vi "LVClass_CorrectionDataManager ComputeDeltaCmdFromDeltaSWithCLSmooth.vi"(0 "CorrectionDataManager in":refnum<class "CorrectionDataManager.lvclass">, 5 "Delta Slopes IN":refnum<class "HasoSlopes.lvclass">, 7 "Gain in":dbl min=0.0 max=1.0, 9 "ClosedLoopSmoothing in":refnum<class "ClosedLoopSmoothing.lvclass">, 11 "error in (no error)":errorcluster, 12 "do tilt check":bool=TRUE) -> (4 "CorrectionDataManager out":refnum<class "CorrectionDataManager.lvclass">, 6 "Delta Slopes OUT":refnum<class "HasoSlopes.lvclass">, 8 "Gain out":dbl min=0.0 max=1.0, 10 "ClosedLoopSmoothing out":refnum<class "ClosedLoopSmoothing.lvclass">, 13 "DeltaPosition":T1, 15 "error out":errorcluster)   [LabVIEW 2020, in "CorrectionDataManager.lvclass"]
doc: "--------------------------------------------------------------------------------\n\n<B>corrdata_managerIn</B> : CorrDataManager object.\n\n<B>corrdata_managerOut</B> : CorrDataManager object.\n\n<B>delta_slopes</B> : Array of target slopes deltas (stored as cHasoSlopes).\n\n<B>gain</B> : Smoothing factor for loop iterations.\n\n<B>delta_Commands</B> : Array of size actuators count, containing the commands deltas (relatives\n variations to apply from actuators initial positions).\n\n<B>min</B> : WavefrontCorrector preferences : lowest command value.\n\n<B>max</B> : WavefrontCorrector preferences : highest command value.\n\n<B>validity</B> : WavefrontCorrector preferences : status.\n\n<B>fixed_values</B> : WavefrontCorrector preferences : fixed positions.\n\n<B>ErrorIn</B> : Error\n\n<B>ErrorOut</B> : Error"
uses:
  CorrectionDataManager.lvclass
  HasoSlopes.lvclass
  Wavefront Corrector Position.ctl
  ClosedLoopSmoothing.lvclass
  CorrectionDataManager.lvclass/CorrectionDataManager.ctl
  LVClass_ClosedLoopSmoothing Read ClosedLoopSmooth.vi
  LVClass_HasoSlopes Read HasoSlopes _ property.vi
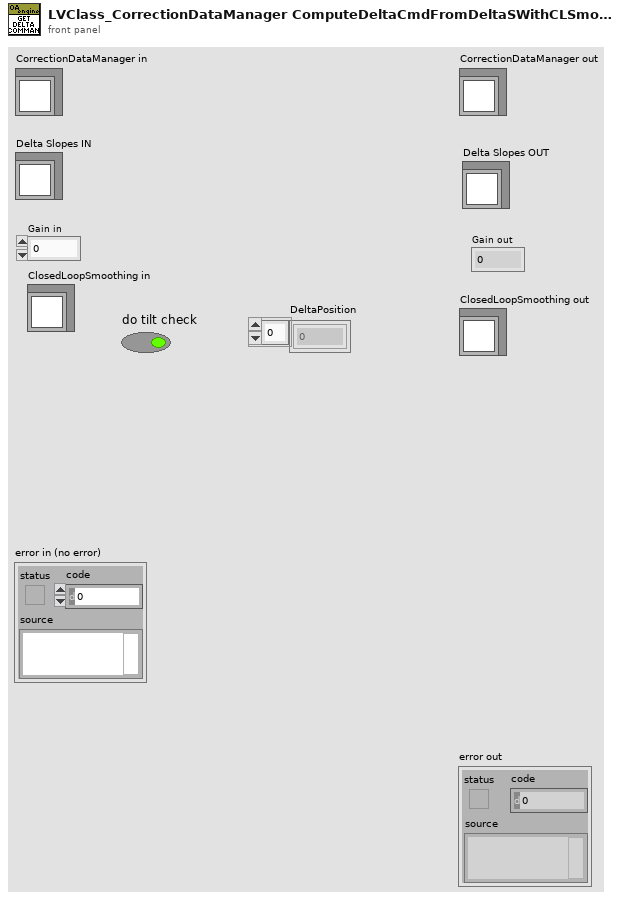
[diagram p1: front panel]
types:
  T1 = typedef "Wavefront Corrector Position.ctl" = sgl[]
  T2 = typedef "Wavefront Corrector states - ONE.ctl" = cluster{"Max":sgl, "Min":sgl, "Validity":enum16{"valid", "fixed", "invalid"}, "Fixed_Position":sgl}
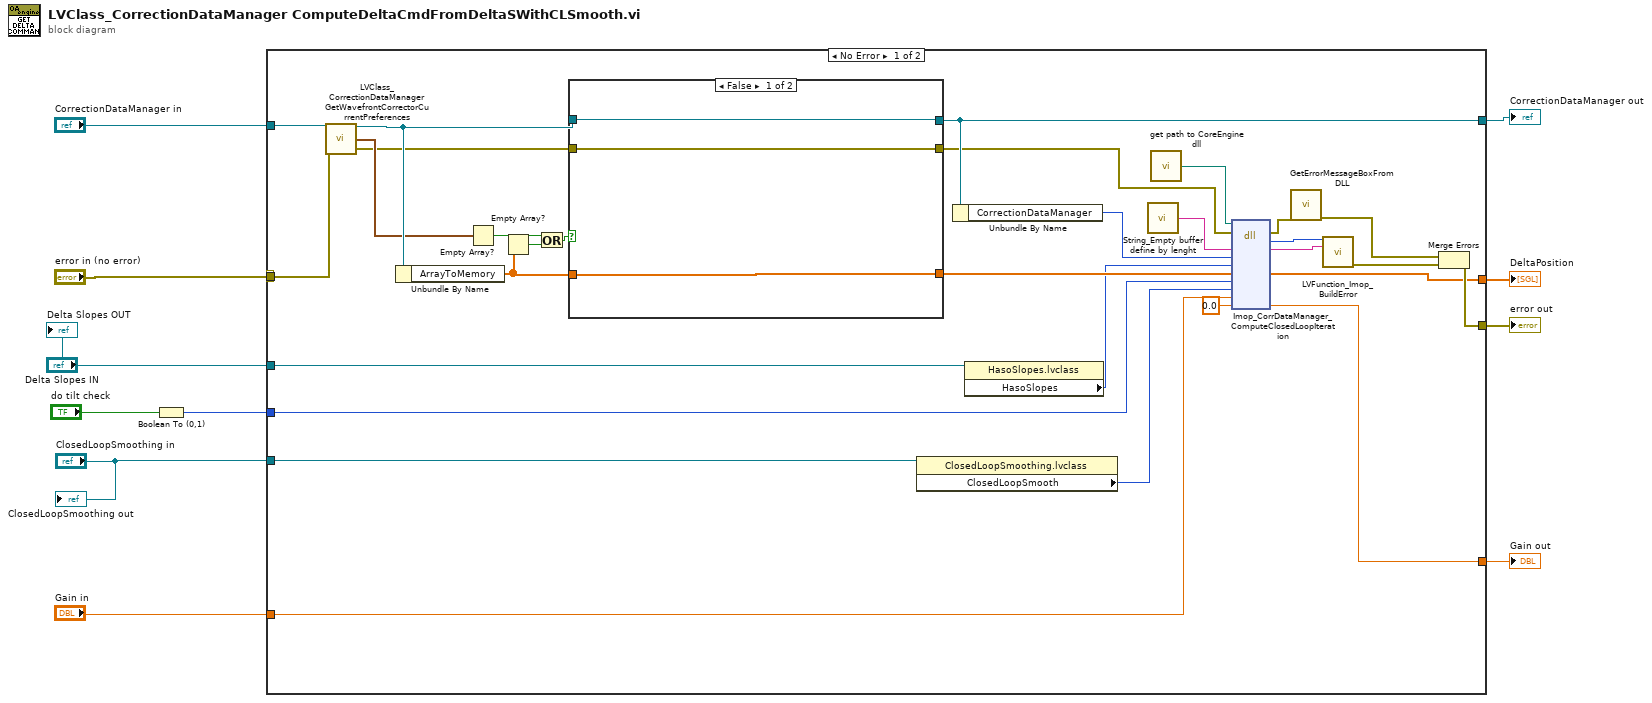
[diagram p0: block diagram]
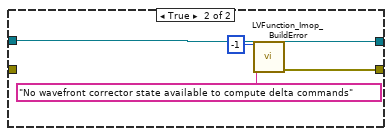
[diagram p2: hidden frame]
diagram:
  n1 = Boolean To (0,1)(Boolean="do tilt check") -> (0, 1=w2:i16)
  n2 = case shown="No Error" "error in (no error)" {
    selector: "error in (no error)" -> [_ w50]
    tunnel: [w34 w50] -> w11
    tunnel: [w15 w49] -> w10
    tunnel: "CorrectionDataManager in" -> [w25 w49]
    tunnel: "Delta Slopes IN" -> [w18 _]
    tunnel: "Gain in" -> [w33 _]
    tunnel: [w32 _] -> w6
    tunnel: "ClosedLoopSmoothing in" -> [w20 _]
    tunnel: [w19 _] -> w4
    tunnel: w2 -> [w16 _]
    tunnel: "error in (no error)" -> [w12 _]
    frame No Error {
      n3 = call "LVClass_CorrectionDataManager GetWavefrontCorrectorCurrentPreferences.vi"("CorrectionDataManager in"=w25, "error in (no error)"=w12) -> ("CorrectionDataManager out"=w24:refnum<class "CorrectionDataManager.lvclass">, "Wavefront Corrector State"=w23:T2[], "error out"=w13:errorcluster)  [unwired: 11 in]
      n4 = Unbundle By Name(w24) -> ("ArrayToMemory"=w26:T1)
      n5 = Empty Array?(array=w23) -> (empty?=w29:bool)
      n6 = Empty Array?(array=w26) -> (empty?=w30:bool)
      n7 = Or(x=w30, y=w29) -> (x .or. y?=w28:bool)
      n8 = case shown="False" w28 {
        tunnel: w24 -> [w43 w48]
        tunnel: [w43 w48] -> w15
        tunnel: [w42 w47] -> w14
        tunnel: [w44 _] -> w27
        tunnel: w26 -> [w44 _]
        tunnel: w13 -> [w42 _]
        frame False {
        }
        frame True {
          n9 = call "LVFunction_Imop_BuildError.vi"("code"=-1, "String to Prepend to source (\"\")"="No wavefront corrector state available to compute delta commands" ("String to Prepend to source (\"\")")) -> ("error out"=w47:errorcluster)  [unwired: 13 in]
        }
      }
      n10 = property class="ClosedLoopSmoothing.lvclass"(reference=w20) -> ("ClosedLoopSmooth"=w21:i32)  [unwired: 1 in, 2 out]
      n11 = Unbundle By Name(w15) -> ("CorrectionDataManager"=w31:i32)
      n12 = property class="HasoSlopes.lvclass"(reference=w18) -> ("HasoSlopes"=w17:i32)  [unwired: 1 in, 2 out]
      n13 = call "String_Empty buffer define by lenght.vi"() -> ("Empty buffer"=w39:string)  [unwired: 1 in]
      n14 = call "get path to CoreEngine dll.vi"() -> ("path to c_interface_vc100.dll"=w38:path)  [unwired: 12 in, 3 out]
      n15 = dll-call lib="D:/FLE/0.Code/CoreEngine4_Suite/LV2011_interface/DLLs/c_interface_vc100.dll" fn="Imop_CorrDataManager_ComputeClosedLoopIteration"(path in=w38, error in=w14, "message"=w39, "WavefrontCorrection"=w31, "deltaHasoSlopes"=w17, "delta_commands"=w27, "do tilt check"=w16, "smoothing_params"=w21, "specified_loop_gain"=w33, "applied_loop_gain"=sgl 0.0) -> (error out=w37:errorcluster, "return type"=w41:i32, "message"=w40:string, "delta_commands"=w32:sgl[], "applied_loop_gain"=w19:sgl)  [unwired: 6 in, 1 out]
      n16 = call "GetErrorMessageBoxFromDLL.vi"("error IN"=w37) -> ("error OUT"=w36:errorcluster)  [unwired: 10 in]
      n17 = call "LVFunction_Imop_BuildError.vi"("code"=w41, "String to Prepend to source (\"\")"=w40) -> ("error out"=w35:errorcluster)  [unwired: 13 in]
      n18 = Merge Errors(w36, w35) -> (w34:errorcluster)
    }
    frame Error {
    }
  }
  "error out" <- w11
  "CorrectionDataManager out" <- w10
  "DeltaPosition" <- w6
  "Gain out" <- w4
  "Delta Slopes OUT" <- "Delta Slopes IN"
  "ClosedLoopSmoothing out" <- "ClosedLoopSmoothing in"
